vi "xiUtils - Cursor Set - Idle.vi"(8 "error in (no error)":errorcluster, 11 "VI reference (Top Level VI)":refnum<vi>) -> (0 "error out":errorcluster)   [LabVIEW 2015]
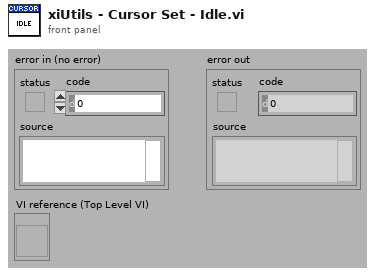
[diagram p1: front panel]
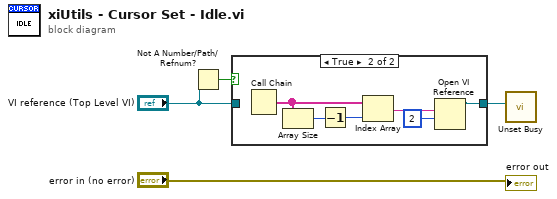
[diagram p0: block diagram]
diagram:
  n1 = Not A Number/Path/Refnum?(number/path/refnum="VI reference (Top Level VI)") -> (NaN/Path/Refnum?=w3:bool)
  n2 = case shown="True" w3 {
    tunnel: "VI reference (Top Level VI)" -> [w5 _]
    tunnel: [w5 w6] -> w1
    frame False {
    }
    frame True {
      n3 = Call Chain() -> (call chain=w8:string[])
      n4 = Array Size(array=w8) -> (size(s)=w9:i32)
      n5 = Decrement(x=w9) -> (x-1=w7:i32)
      n6 = Index Array(array=w8, index=w7) -> (element=w11:string)
      n7 = Open VI Reference(vi path=w11, options=2 ("0x02 =>\nOpen Templates for Editing.  If called by a template, then need template reference.")) -> (vi reference=w6:refnum<vi>)  [unwired: 4 in, 1 out]
    }
  }
  n8 = call <vilib>:"Unset Busy.vi"("VI reference (current VI)"=w1) -> ()  [unwired: 10 in, 1 out]
  "error out" <- "error in (no error)"
